vi "marks_report.vi"   [LabVIEW 2014]
uses:
  <vilib>/addons/_office/_exclsub.llb/font.ctl
  <vilib>/addons/_office/excel.llb/Excel Get Data (dbl).vi
  <vilib>/addons/_office/excel.llb/Excel Get Data (str).vi
  <vilib>/Analysis/Matrix/Numeric/Conversions/Array To Matrix - RA2.vi
  <vilib>/addons/_office/excel.llb/Excel Easy Table (num).vi
  <vilib>/Utility/NIReport.llb/NI_report.lvclass
  <vilib>/addons/_office/NI_ReportGenerationToolkit.lvlib
  <vilib>/Utility/NIReport.llb/Excel/NI_Excel.lvclass
  <vilib>/Analysis/Matrix/NI_Matrix.lvlib
types:
  T1 = cluster{"on/off":bool, "weight":i32, "color":u32}
  T2 = typedef "NI_ReportGenerationToolkit.lvlib/font.ctl" = cluster{"font name":string, "font size":dbl, "bold":u16, "italic":u16, "underline":u16, "strike through":u16, "font color":u32}
  T3 = enum16{"Standard Report", "HTML", "Word", "Excel"}
  T4 = typedef "NI_Matrix.lvlib/RealMatrix.ctl" = dbl[][]
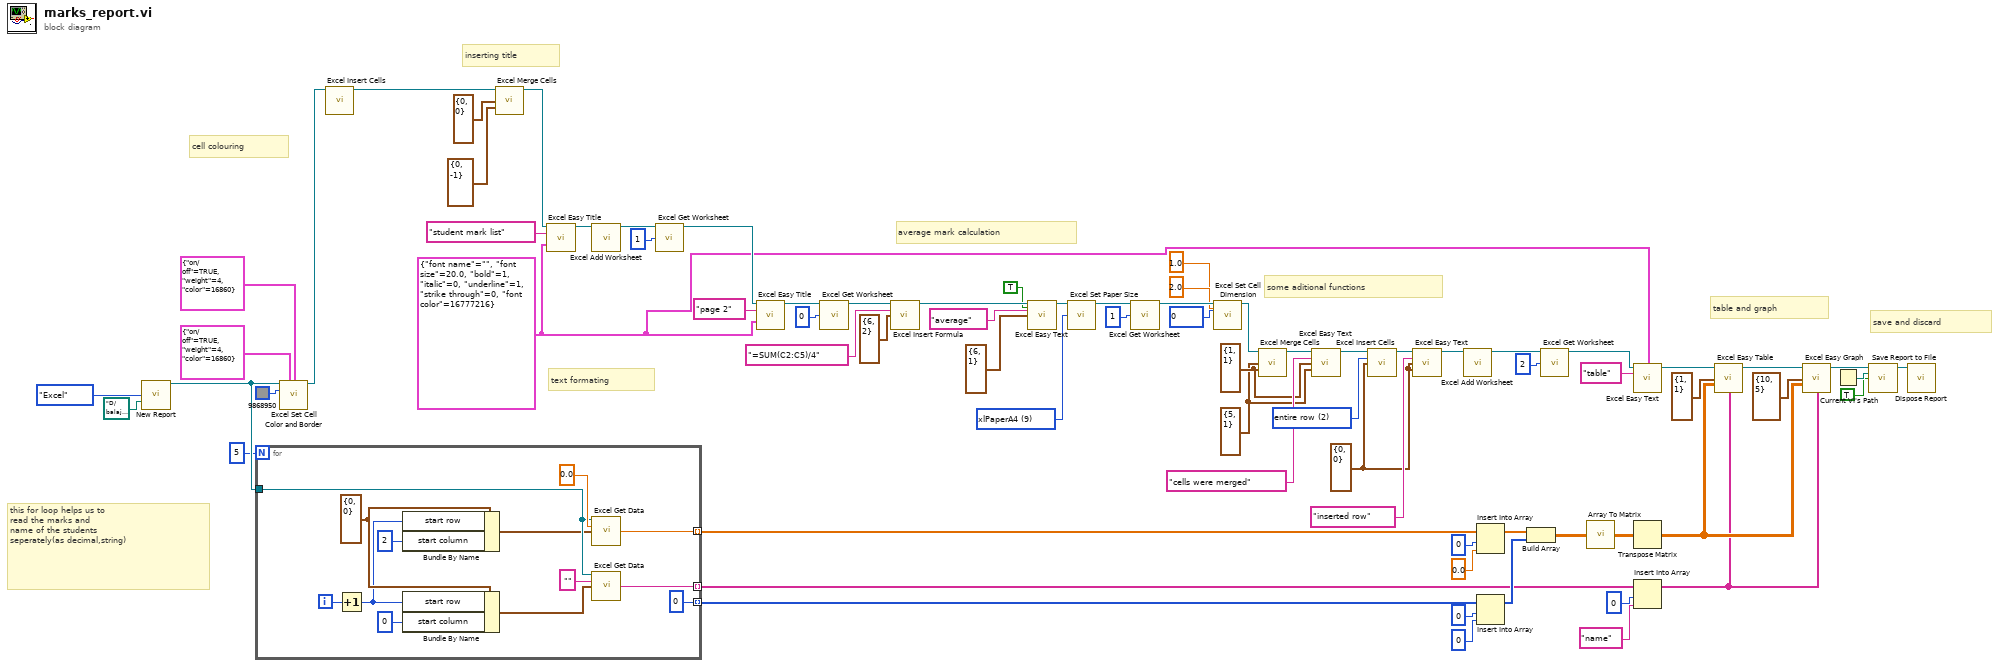
[diagram p0: block diagram]
diagram:
  w32 = cluster{"row":i32, "column":i32} {"row"=0, "column"=0} ("start (0, 0)")
  w35 = u16 2 items=["shift cells right", "shift cells down", "entire row", "entire column"] ("mode (entire row)")
  w38 = cluster{"row":i32, "column":i32} {"row"=1, "column"=1} ("end (-1, -1)")
  w37 = cluster{"row":i32, "column":i32} {"row"=5, "column"=1} ("start (-1, -1)")
  w49 = 9 items=["xlPaper10x14"=16, "xlPaper11x17"=17, "xlPaperA3"=8, "xlPaperA4"=9, "xlPaperA4Small"=10, "xlPaperA5"=11, "xlPaperB4"=12, "xlPaperB5"=13, "xlPaperCsheet"=24, "xlPaperDsheet"=25, "xlPaperEnvelope10"=20, "xlPaperEnvelope11"=21, "xlPaperEnvelope12"=22, "xlPaperEnvelope14"=23, "xlPaperEnvelope9"=19, "xlPaperEnvelopeB4"=33, "xlPaperEnvelopeB5"=34, "xlPaperEnvelopeB6"=35, "xlPaperEnvelopeC3"=29, "xlPaperEnvelopeC4"=30, "xlPaperEnvelopeC5"=28, "xlPaperEnvelopeC6"=31, "xlPaperEnvelopeC65"=32, "xlPaperEnvelopeDL"=27, "xlPaperEnvelopeItaly"=36, "xlPaperEnvelopeMonarch"=37, "xlPaperEnvelopePersonal"=38, "xlPaperEsheet"=26, "xlPaperExecutive"=7, "xlPaperFanfoldLegalGerman"=41, "xlPaperFanfoldStdGerman"=40, "xlPaperFanfoldUS"=39, "xlPaperFolio"=14, "xlPaperLedger"=4, "xlPaperLegal"=5, "xlPaperLetter"=1, "xlPaperLetterSmall"=2, "xlPaperNote"=18, "xlPaperQuarto"=15, "xlPaperStatement"=6, "xlPaperTabloid"=3, "xlPaperUser"=256] ("paper size (letter)")
  w1 = T2 {"font name"="", "font size"=20.0, "bold"=1, "italic"=0, "underline"=1, "strike through"=0, "font color"=16777216} ("font")
  # "text formating"
  # "inserting title"
  # "cell colouring"
  # "save and discard"
  # "table and graph"
  # "some aditional functions"
  # "average mark calculation"
  # "this for loop helps us to\nread the marks and\nname of the students\nseperately(as decimal,string)"
  n1 = call <vilib>:"New Report.vi"("report type"=T3."Excel", "template (empty)"=path "D:/balaji_doc/vi_files/reprort_proj/report_generation_toolkit.xlsx" ("file path (dialog if empty)")) -> ("report out"=w31:refnum<class "NI_report.lvclass">)  [unwired: 12 in, 1 out]
  n2 = for {
    N: 5 -> [_]
    tunnel: w31 -> [w82]
    tunnel: [w78] -> w13 mode=indexing
    tunnel: [w76] -> w8 mode=indexing
    tunnel: [0] -> w17 mode=indexing
    i -> [w84]
    w81 = cluster{"start row":i32, "start column":i32} {"start row"=0, "start column"=0} ("start (0, 0)")
    n3 = Increment(x=w84) -> (x+1=w80:i32)
    n4 = Bundle By Name(cluster=w81, "start row"=w80, "start column"=2) -> (w77:cluster{"start row":i32, "start column":i32})
    n5 = Bundle By Name(cluster=w81, "start row"=w80, "start column"=0) -> (w87:cluster{"start row":i32, "start column":i32})
    n6 = call-poly <vilib>:"Excel Get Data.vi"("report in"=w82, "data type"=0.0 ("Numeric"), "start (0, 0)"=w77) -> ("data"=w78:dbl)  [unwired: 10 in, 2 out]
    n7 = call-poly <vilib>:"Excel Get Data.vi"("report in"=w82, "data type"="", "start (0, 0)"=w87) -> ("data"=w76:string)  [unwired: 10 in, 2 out]
  }
  n8 = call <vilib>:"Excel Set Cell Color and Border.vi"("report in"=w31, "inside border"=T1 {"on/off"=TRUE, "weight"=4, "color"=16860}, "outside border"=T1 {"on/off"=TRUE, "weight"=4, "color"=16860}, "background color (w)"=u32 9868950) -> ("report out"=w46:refnum<class "NI_report.lvclass">)  [unwired: 10 in, 1 out]
  n9 = call <vilib>:"Excel Insert Cells.vi"("report in"=w46) -> ("report out"=w63:refnum<class "NI_report.lvclass">)  [unwired: 13 in, 1 out]
  n10 = call <vilib>:"Excel Merge Cells.vi"("report in"=w63, "start (-1, -1)"=cluster{"row":i32, "column":i32} {"row"=0, "column"=0}, "end (-1, -1)"=cluster{"row":i32, "column":i32} {"row"=0, "column"=-1}) -> ("report out"=w60:refnum<class "NI_report.lvclass">)  [unwired: 11 in, 1 out]
  n11 = call <vilib>:"Excel Easy Title.vi"("report in"=w60, "title"="student mark list", "font"=w1) -> ("report out"=w71:refnum<class "NI_report.lvclass">)  [unwired: 10 in, 2 out]
  n12 = call <vilib>:"Excel Add Worksheet.vi"("report in"=w71) -> ("report out"=w70:refnum<class "NI_report.lvclass">)  [unwired: 13 in, 1 out]
  n13 = call <vilib>:"Excel Get Worksheet.vi"("report in"=w70, "worksheet index (0)"=1) -> ("report out"=w68:refnum<class "NI_report.lvclass">)  [unwired: 12 in, 1 out]
  n14 = call <vilib>:"Excel Easy Title.vi"("report in"=w68, "title"="page 2", "font"=w1) -> ("report out"=w56:refnum<class "NI_report.lvclass">)  [unwired: 10 in, 2 out]
  n15 = call <vilib>:"Excel Get Worksheet.vi"("report in"=w56, "worksheet index (0)"=0) -> ("report out"=w55:refnum<class "NI_report.lvclass">)  [unwired: 12 in, 1 out]
  n16 = call <vilib>:"Excel Insert Formula.vi"("report in"=w55, "formula"="=SUM(C2:C5)/4", "start (0, 0)"=cluster{"row":i32, "column":i32} {"row"=6, "column"=2}) -> ("report out"=w54:refnum<class "NI_report.lvclass">)  [unwired: 11 in, 1 out]
  n17 = call <vilib>:"Excel Easy Text.vi"("report in"=w54, "border? (F)"=TRUE, "text"="average", "start (-1, -1)"=cluster{"row":i32, "column":i32} {"row"=6, "column"=1}) -> ("report out"=w50:refnum<class "NI_report.lvclass">)  [unwired: 7 in, 4 out]
  n18 = call <vilib>:"Excel Set Paper Size.vi"("report in"=w50, "paper size (letter)"=w49) -> ("report out"=w47:refnum<class "NI_report.lvclass">)  [unwired: 12 in, 1 out]
  n19 = call <vilib>:"Excel Get Worksheet.vi"("report in"=w47, "worksheet index (0)"=1) -> ("report out"=w45:refnum<class "NI_report.lvclass">)  [unwired: 12 in, 1 out]
  n20 = call <vilib>:"Excel Set Cell Dimension.vi"("report in"=w45, "width (-1)"=2.0, "height (-1)"=1.0, "measurement system"=u16 0) -> ("report out"=w41:refnum<class "NI_report.lvclass">)  [unwired: 10 in, 1 out]
  n21 = call <vilib>:"Excel Merge Cells.vi"("report in"=w41, "start (-1, -1)"=w37, "end (-1, -1)"=w38) -> ("report out"=w40:refnum<class "NI_report.lvclass">)  [unwired: 11 in, 1 out]
  n22 = call <vilib>:"Excel Easy Text.vi"("report in"=w40, "text"="cells were merged", "start (-1, -1)"=w38, "end (-1, -1)"=w37) -> ("report out"=w36:refnum<class "NI_report.lvclass">)  [unwired: 7 in, 4 out]
  n23 = call <vilib>:"Excel Insert Cells.vi"("report in"=w36, "mode (entire row)"=w35, "start (0, 0)"=w32) -> ("report out"=w34:refnum<class "NI_report.lvclass">)  [unwired: 11 in, 1 out]
  n24 = call <vilib>:"Excel Easy Text.vi"("report in"=w34, "text"="inserted row", "start (-1, -1)"=w32, "end (-1, -1)"=w32) -> ("report out"=w27:refnum<class "NI_report.lvclass">)  [unwired: 7 in, 4 out]
  n25 = call <vilib>:"Excel Add Worksheet.vi"("report in"=w27) -> ("report out"=w25:refnum<class "NI_report.lvclass">)  [unwired: 13 in, 1 out]
  n26 = Insert Into Array(array=w13, index=0, new element=0.0 ("new element/subarray")) -> (w10:dbl[])
  n27 = Insert Into Array(array=w17, index=0, new element=0 ("new element/subarray")) -> (w14:i32[])
  n28 = Build Array(w10, w14) -> (w29:dbl[][])
  n29 = call <vilib>:"Excel Get Worksheet.vi"("report in"=w25, "worksheet index (0)"=2) -> ("report out"=w23:refnum<class "NI_report.lvclass">)  [unwired: 12 in, 1 out]
  n30 = call-poly <vilib>:"Array To Matrix.vi"("Real 2D Array"=w29) -> ("Real Matrix"=w28:T4)
  n31 = call <vilib>:"Excel Easy Text.vi"("report in"=w23, "font"=w1, "text"="table") -> ("report out"=w22:refnum<class "NI_report.lvclass">)  [unwired: 8 in, 4 out]
  n32 = Transpose Matrix(1:w28) -> (0:w18:T4)
  n33 = Insert Into Array(array=w8, index=0, new element="name" ("new element/subarray")) -> (w9:string[])
  n34 = call-poly <vilib>:"Excel Easy Table.vi"("report in"=w22, "start (0, 0)"=cluster{"row":i32, "column":i32} {"row"=1, "column"=1}, "text data"=w18, "row headers"=w9) -> ("report out"=w21:refnum<class "NI_report.lvclass">)  [unwired: 7 in, 4 out]
  n35 = call <vilib>:"Excel Easy Graph.vi"("report in"=w21, "start (0, 0)"=cluster{"row":i32, "column":i32} {"row"=10, "column"=5}, "data"=w18, "row headers"=w9) -> ("report out"=w5:refnum<class "NI_report.lvclass">)  [unwired: 10 in, 1 out]
  n36 = Current VI's Path() -> (path=w4:path)
  n37 = call-dynamic "Save Report to File.vi"("report in"=w5, "report file path"=w4, "prompt to replace? (F)"=TRUE) -> ("report out"=w2:refnum<class "NI_report.lvclass">)  [unwired: 11 in, 1 out]
  n38 = call-dynamic "Dispose Report.vi"("report in"=w2) -> ()  [unwired: 14 in, 1 out]
